vi "MB Serial Master Query.vi"(4 "Timeout":u32=10000, 6 "Serial Parameters":T1 {"Slave Address" format="%.0x"}, 7 "Modbus Data Unit In":T3={"Function Code"=1, "Data"=[]} {"Function Code" items=["Read Coils"=1, "Read Discrete Inputs"=2, "Read Holding Registers"=3, "Read Input Registers"=4, "Write Single Coil"=5, "Write Single Register"=6, "Read Exception Status"=7, "Write Multiple Coils"=15, "Write Multiple Registers"=16]; "Data" format="%.0x"}, 8 "error in (no error)":errorcluster, 9 "Use MODBUS Data Unit?":bool, 10 "Modbus Command":T2={"Function Code"=1, "Starting Address"=0, "Quantity"=0, "Data"=[], "Discrete"=[]} {"Function Code" items=["Read Coils"=1, "Read Discrete Inputs"=2, "Read Holding Registers"=3, "Read Input Registers"=4, "Write Single Coil"=5, "Write Single Register"=6, "Read Exception Status"=7, "Write Multiple Coils"=15, "Write Multiple Registers"=16]}, 11 "VISA resource name":refnum<visa-resource-name>) -> (0 "error out":errorcluster, 1 "Exception Code":u8 format="%.0x", 2 "Registers":cluster{"Registers":u16[], "Discrete":bool[]}, 3 "VISA resource name out":refnum<visa-resource-name>, 5 "Modbus Data Unit Out":T3={"Function Code"=1, "Data"=[]} {"Function Code" items=["Read Coils"=1, "Read Discrete Inputs"=2, "Read Holding Registers"=3, "Read Input Registers"=4, "Write Single Coil"=5, "Write Single Register"=6, "Read Exception Status"=7, "Write Multiple Coils"=15, "Write Multiple Registers"=16]; "Data" format="%.0x"})   [LabVIEW 2011]
uses:
  MB Modbus Data Unit.ctl
  MB Modbus Command.ctl
panel:
  # "VI Name: MB Serial Master Query.vi\nPurpose: Performs a Modbus query.\nReentrant."
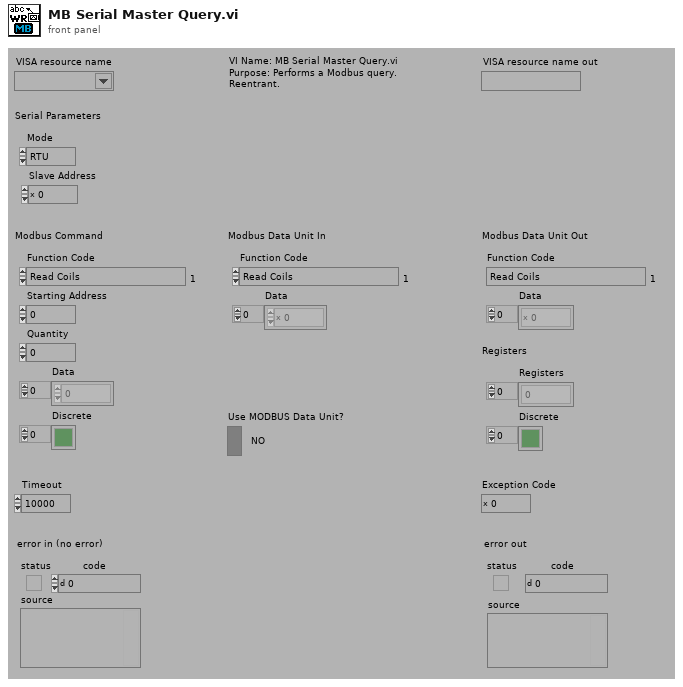
[diagram p1: front panel]
types:
  T1 = cluster{"Mode":enum16{"RTU", "ASCII"}, "Slave Address":u8}
  T2 = typedef "MB Modbus Command.ctl" = cluster{"Function Code":u8, "Starting Address":u16, "Quantity":u16, "Data":u16[], "Discrete":bool[]}
  T3 = typedef "MB Modbus Data Unit.ctl" = cluster{"Function Code":u8, "Data":u8[]}
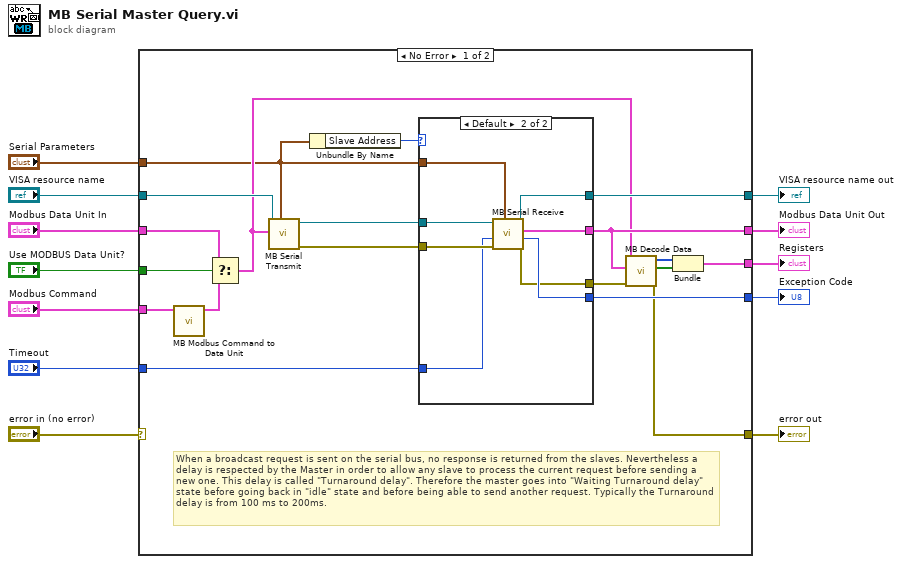
[diagram p0: block diagram]
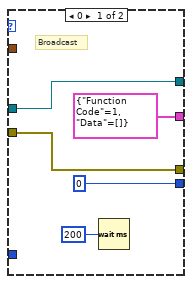
[diagram p2: hidden frame]
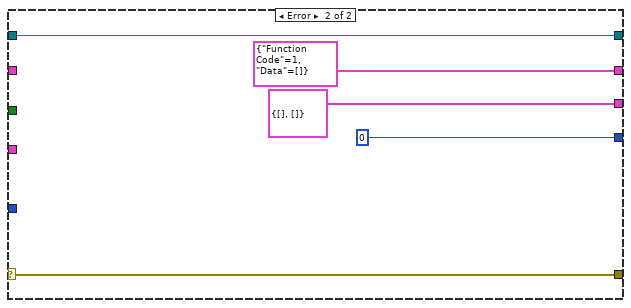
[diagram p3: hidden frame]
diagram:
  n1 = case shown="No Error" "error in (no error)" {
    selector: "error in (no error)" -> [_ w45]
    tunnel: [w24 T3 {"Function Code"=1, "Data"=[]} ("MODBUS Data Unit")] -> w5
    tunnel: [w28 u8 0 ("Exception Code")] -> w12
    tunnel: [w22 w45] -> w3
    tunnel: "VISA resource name" -> [w31 w49]
    tunnel: "Timeout" -> [w30 _]
    tunnel: [w29 w49] -> w9
    tunnel: "Modbus Data Unit In" -> [w27 _]
    tunnel: "Use MODBUS Data Unit?" -> [w26 _]
    tunnel: "Modbus Command" -> [w25 _]
    tunnel: [w23 cluster{"Registers":u16[], "Discrete":bool[]} {"Registers"=[], "Discrete"=[]}] -> w4
    tunnel: "Serial Parameters" -> [w13 _]
    frame No Error {
      # "When a broadcast request is sent on the serial bus, no response is returned from the slaves. Nevertheless a delay is respected by the Master in order to allow any slave to process the current request before sending a new one. This delay is called \"Turnaround delay\". Therefore the master goes into \"Waiting Turnaround delay\" state before going back in \"idle\" state and before being able to send another request. Typically the Turnaround delay is from 100 ms to 200ms."
      n2 = call "MB Modbus Command to Data Unit.vi"("Modbus Command"=w25) -> ("Modbus Data Unit"=w18:T3)  [unwired: 10 out]
      n3 = Select(t=w27, s=w26, f=w18) -> (s? t:f=w14:T3)
      n4 = call "MB Serial Transmit.vi"("Serial Parameters"=w13, "Modbus Data Unit"=w14, "VISA resource name"=w31) -> ("error out"=w20:errorcluster, "VISA resource name out"=w21:refnum<visa-resource-name>)  [unwired: 3 in, 4 out]
      n5 = Unbundle By Name(w13) -> ("Slave Address"=w19:u8)
      n6 = case shown="Default" w19 {
        tunnel: w21 -> [w36 w44]
        tunnel: w20 -> [w33 w43]
        tunnel: w30 -> [_ w42]
        tunnel: w13 -> [_ w41]
        tunnel: [w36 w40] -> w29
        tunnel: [u8 0 ("Exception Code") w39] -> w28
        tunnel: [T3 {"Function Code"=1, "Data"=[]} ("MODBUS Data Unit") w38] -> w24
        tunnel: [w33 w37] -> w17
        frame 0 {
          # "Broadcast"
          n7 = Wait (ms)(milliseconds to wait=u32 200) -> ()  [unwired: 1 out]
        }
        frame Default {
          n8 = call "MB Serial Receive.vi"("Serial Parameters"=w41, "error in (no error)"=w43, "Timeout"=w42, "VISA resource name"=w44) -> ("error out"=w37:errorcluster, "Exception Code"=w39:u8, "Modbus Data Unit"=w38:T3, "VISA resource name out"=w40:refnum<visa-resource-name>)  [unwired: 1 in, 3 out]
        }
      }
      n9 = call "MB Decode Data.vi"("error in (no error)"=w17, "Response MDU"=w24, "Request MDU"=w14) -> ("error out"=w22:errorcluster, "Discrete"=w15:bool[], "Registers"=w16:u16[])  [unwired: 6 out]
      n10 = Bundle("Registers"=w16, "Discrete"=w15) -> (w23:cluster{"Registers":u16[], "Discrete":bool[]})  [unwired: 1 out]
    }
    frame Error {
    }
  }
  "error out" <- w3
  "Exception Code" <- w12
  "VISA resource name out" <- w9
  "Modbus Data Unit Out" <- w5
  "Registers" <- w4
